vi "Generate Digital Pulse.vi"(8 "error in (no error)":errorcluster, 10 "Channel":string="Aliases/Counter Writer", 11 "WorkspaceManager":T1) -> (0 "error out":errorcluster, 3 "Workspace Manager out":T1)   [LabVIEW 2026, in "Scan Engine Specialty Digital System Tests.lvclass"]
uses:
  Scan Engine Specialty Digital System Tests.lvclass
  <vilib>/NI/VeriStand Custom Device Testing Tools/VeriStandTestUtilities/VeriStandTestUtilities.lvlib
  NationalInstruments.VeriStand.ClientAPI
  <vilib>/NI VeriStand/Execution/Workspace/WorkspaceAPI.ctl
  <vilib>/NI VeriStand/Execution/Workspace/NI_VS Workspace ExecutionAPI.lvlib
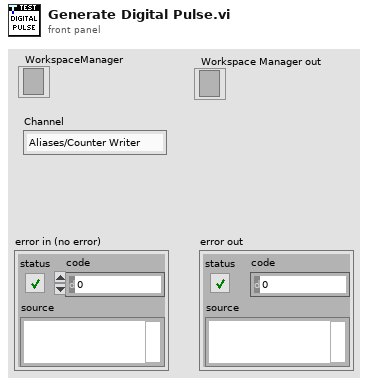
[diagram p1: front panel]
types:
  T1 = typedef "NI_VS Workspace ExecutionAPI.lvlib/WorkspaceAPI.ctl" = refnum<k24>
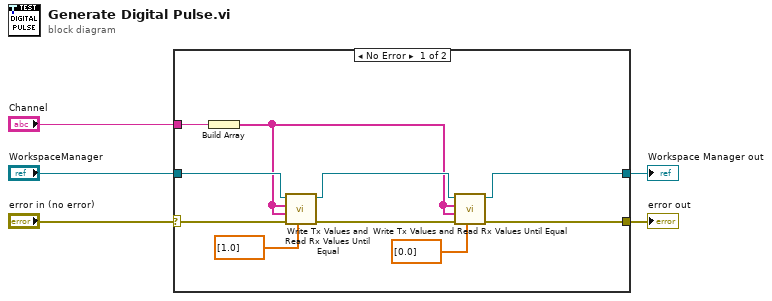
[diagram p0: block diagram]
diagram:
  n1 = case shown="No Error" "error in (no error)" {
    selector: "error in (no error)" -> [w13 w17]
    tunnel: "Channel" -> [w15 _]
    tunnel: [w14 w16] -> w4
    tunnel: [w10 w17] -> w3
    tunnel: "WorkspaceManager" -> [w11 w16]
    frame No Error {
      n2 = Build Array(w15) -> (w8:string[])
      n3 = call <vilib>:"Write Tx Values and Read Rx Values Until Equal.vi"("Tx values"=dbl[] [1.0], "error in"=w13, "Rx aliases"=w8, "Tx aliases"=w8, "workspace manager in"=w11) -> ("error out"=w9:errorcluster, "workspace manager out"=w12:T1)  [unwired: 4 in, 1 out]
      n4 = call <vilib>:"Write Tx Values and Read Rx Values Until Equal.vi"("Tx values"=dbl[] [0.0], "error in"=w9, "Rx aliases"=w8, "Tx aliases"=w8, "workspace manager in"=w12) -> ("error out"=w10:errorcluster, "workspace manager out"=w14:T1)  [unwired: 4 in, 1 out]
    }
    frame Error {
    }
  }
  "Workspace Manager out" <- w4
  "error out" <- w3
